vi "AccDataToRealValue.vi"(11 "Input":i32) -> (3 "output":dbl)   [LabVIEW 2015]
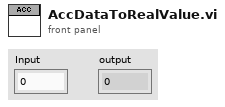
[diagram p1: front panel]
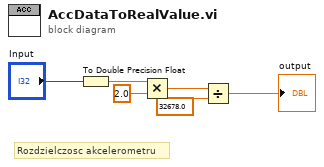
[diagram p0: block diagram]
diagram:
  # "Rozdzielczosc akcelerometru"
  n1 = To Double Precision Float(number="Input") -> (double precision float=w5:dbl)
  n2 = Multiply(x=w5, y=2.0) -> (x*y=w3:dbl)
  n3 = Divide(x=w3, y=32678.0) -> (x/y=→"output":dbl)
